vi "Initialize Registry.vi"(8 "error in (no error)":errorcluster) -> (0 "error out":errorcluster, 3 "Registry out":refnum<class "Registry.lvclass">)   [LabVIEW 2020, in "BCI-1553 API.lvlib" / "Registry.lvlib" / "Registry.lvclass"]
doc: "Creates an instance of the Registry."
uses:
  Registry.lvclass
  Registry.lvclass/Registry.ctl
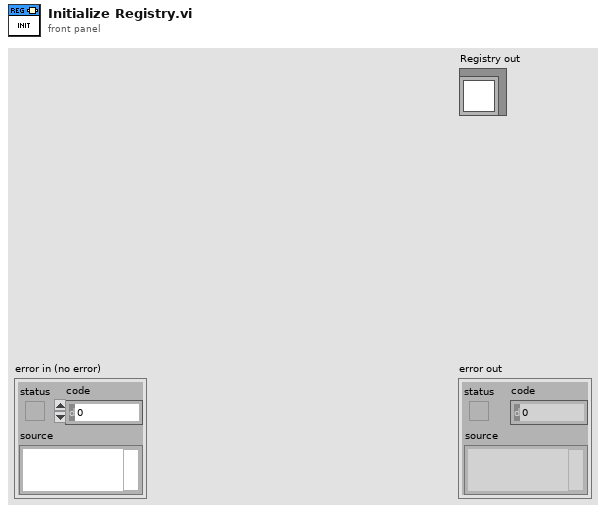
[diagram p1: front panel]
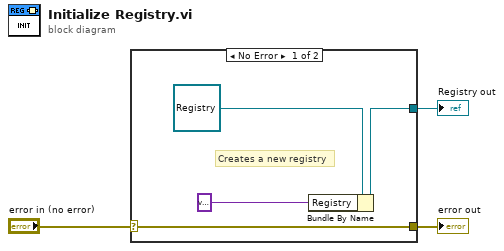
[diagram p0: block diagram]
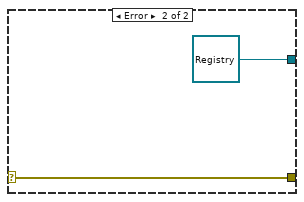
[diagram p2: hidden frame]
diagram:
  n1 = case shown="No Error" "error in (no error)" {
    selector: "error in (no error)" -> [w4 w9]
    tunnel: [w4 w9] -> w2
    tunnel: [w7 refnum<class "Registry.lvclass"> refnum ("Registry in")] -> w1
    frame No Error {
      # "Creates a new registry"
      n2 = Bundle By Name(cluster=refnum<class "Registry.lvclass"> refnum ("Registry in"), "Registry"=variant) -> (w7:refnum<class "Registry.lvclass">)
    }
    frame Error {
    }
  }
  "error out" <- w2
  "Registry out" <- w1
